vi "Main Page.vi"(8 "error in (no error)":errorcluster, 11 "Node Ptr":T2 format="%.0x") -> (0 "error out":errorcluster)   [LabVIEW 2019, in "OPC UA Client Addon System Explorer.lvlib"]
uses:
  OPC UA Client Addon System Explorer.lvlib
  <vilib>/NI VeriStand/Custom Device API/Custom Device Item Ref.ctl
  Addon Shared/Types/OPCConnection.Properties.ctl
  Addon Shared/SubVIs/Constants.vi
  <vilib>/NI VeriStand/Custom Device API/NI VeriStand - Get Item Property.vi
  <vilib>/NI VeriStand/Custom Device API/Get Item Property (String).vi
  <vilib>/NI VeriStand/Custom Device API/Get Item Property (U16).vi
  <vilib>/NI VeriStand/Custom Device API/Get Item Property (Dependent File).vi
  <vilib>/NI VeriStand/Custom Device API/NI VeriStand - Set Item Property.vi
  <vilib>/NI VeriStand/Custom Device API/Set Item Property (String).vi
  <vilib>/NI VeriStand/Custom Device API/Set Item Property (U16).vi
  <vilib>/Utility/libraryn.llb/Get File Extension.vi
  <vilib>/Utility/MD5Checksum.llb/MD5Checksum File.vi
  <vilib>/NI VeriStand/Custom Device API/Set Item Property (Dependent File).vi
  <vilib>/Utility/libraryn.llb/Check if File or Folder Exists.vi
  <vilib>/NI VeriStand/Custom Device API/NI VeriStand - Remove Item Property.vi
  <vilib>/NI VeriStand/Custom Device API/Custom Device API.lvlib
  Addon Shared/OPC UA Client Addon Shared.lvlib
panel:
  out "Version":string
  in  "Header 2":cluster{"Section Name":string}={"Section Name"="Connection Settings"}
  in  "Login Info":cluster{"User Name":string, "Password":string}
  in  "Security Policy":T1
  in  "Server Certificate":path
  in  "Client Certificate":path
  in  "Server Port":u16=49350
  in  "Server IP Address":string
  in  "SHDocVw.IWebBrowser":refnum<k7>(container)
  in  "Header":cluster{"Section Name":string}={"Section Name"="Custom Device Item Settings"}
  in  "Description":string
  in  "Name":string
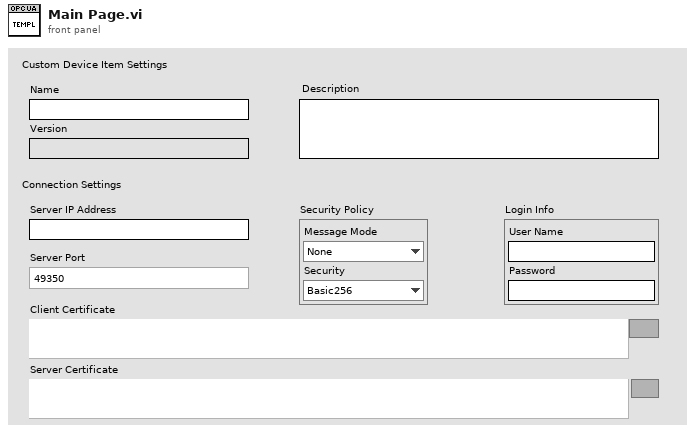
[diagram p1: front panel]
types:
  T1 = cluster{"Message Mode":enum16{"None", "Sign", "Sign and Encrypt"}, "Security":enum16{"Basic256", "Basic128Rsa15"}}
  T2 = typedef "Custom Device API.lvlib/Custom Device Item Ref.ctl" = u64
  T3 = typedef "Custom Device API.lvlib/Custom Device Item Info.ctl" = cluster{"Name":string, "Is Channel":bool, "GUID":string, "Is Waveform":bool}
  T4 = typedef "OPC UA Client Addon Shared.lvlib/OPCConnection.Properties.ctl" = cluster{"Server IP Address":string, "Server Port":u16, "Message Mode":enum16{"None", "Sign", "Sign and Encrypt"}, "Security":enum16{"Basic256", "Basic128Rsa15"}, "User Name":string, "Password":string, "Client Certificate":path, "Server Certificate":path, "Server Certificate (RT)":path, "Client Certificate (RT)":path}
  T5 = typedef "Custom Device API.lvlib/Custom Device Commands.ctl" = enum16{"Default", "Item renamed", "Shutdown", "Dynamic button pressed"}
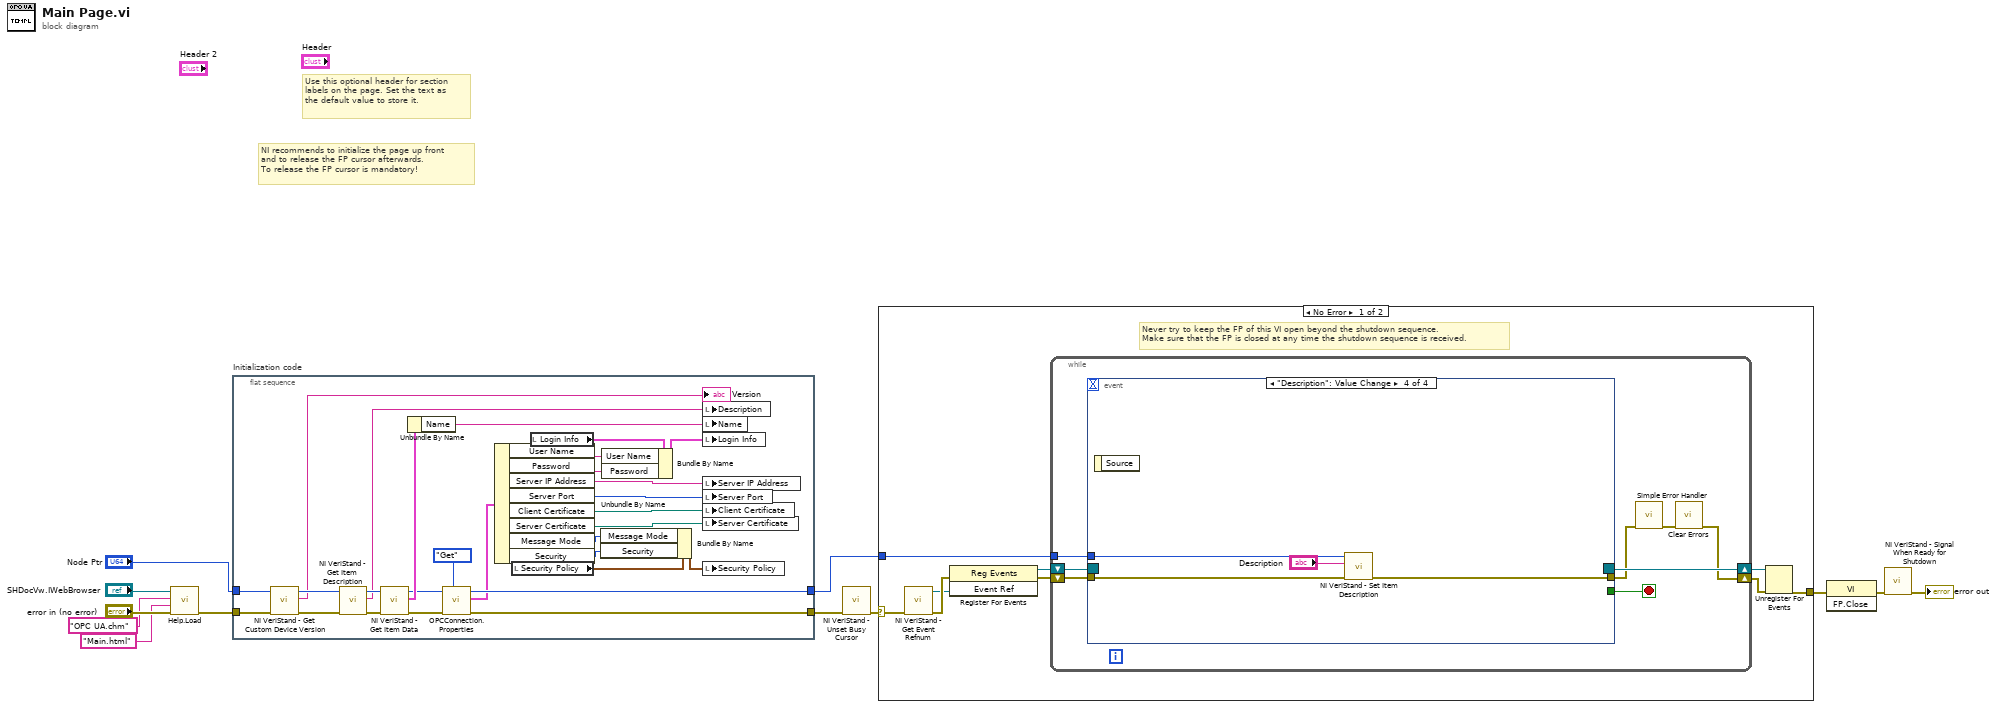
[diagram p0: block diagram]
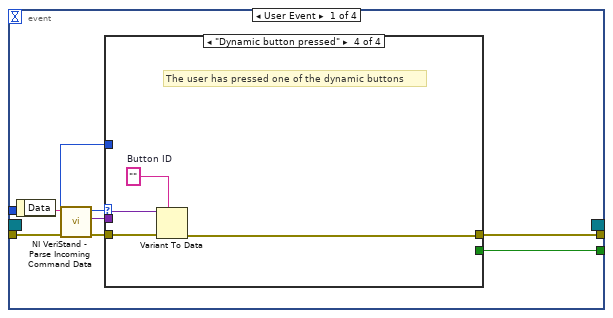
[diagram p2: hidden frame]
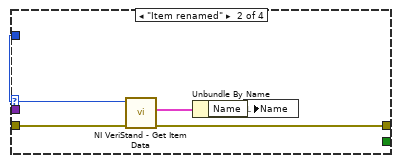
[diagram p4: hidden frame]
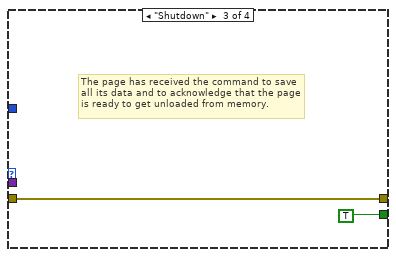
[diagram p5: hidden frame]
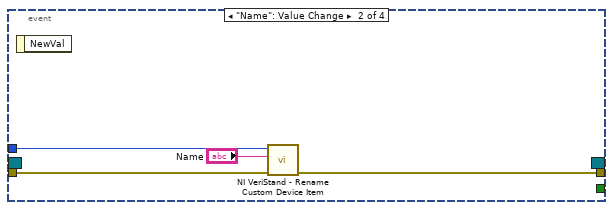
[diagram p6: hidden frame]
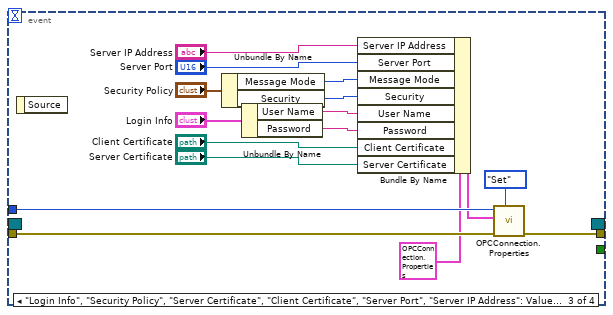
[diagram p7: hidden frame]
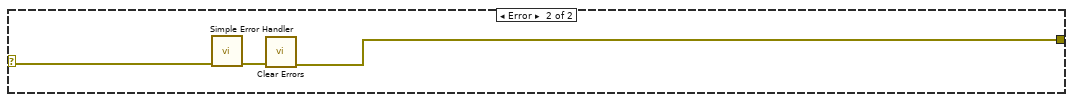
[diagram p8: hidden frame]
diagram:
  # "Use this optional header for section labels on the page. Set the text as the default value to store it."
  # "NI recommends to initialize the page up front\nand to release the FP cursor afterwards.\nTo release the FP cursor is mandatory!"
  n1 = call "Help.Load.vi"("error in (no error)"="error in (no error)", "HTML File"="Main.html" ("Main CHM File"), "Main CHM File"="OPC UA.chm", "SHDocVw.IWebBrowser2"="SHDocVw.IWebBrowser") -> ("error out"=w4:errorcluster)  [unwired: 7 in]
  n2 = flat-sequence "Initialization code" {
    tunnel: w4 -> [w16]
    tunnel: "Node Ptr" -> [w14]
    tunnel: [w33] -> w8
    tunnel: [w31] -> w6
    frame #0 {
      n3 = call <vilib>:"NI VeriStand - Get Custom Device Version.vi"("error in (no error)"=w16, "Device Ref in"=w14) -> ("error out"=w17:errorcluster, "Value"=→"Version":string, "Device Ref out"=w15:T2)  [unwired: 7 in]
      n4 = call <vilib>:"NI VeriStand - Get Item Description.vi"("error in (no error)"=w17, "Item Ref in"=w15) -> ("error out"=w38:errorcluster, "Description"=w39:string, "Item Ref out"=w40:T2)  [unwired: 7 out]
      n5 = call <vilib>:"NI VeriStand - Get Item Data.vi"("error in (no error)"=w38, "Item Ref in"=w40) -> ("error out"=w34:errorcluster, "Item Info"=w37:T3, "Item Ref out"=w32:T2)  [unwired: 7 out]
      n6 = Unbundle By Name(w37) -> ("Name"=w36:string)
      n7 = call "OPCConnection.Properties.vi"("Action"=enum8{"Get", "Set"}."Get", "error in (no error)"=w34, "Item Ref in"=w32) -> ("error out"=w33:errorcluster, "Connection.Properties"=w30:T4, "Item Ref out"=w31:T2)  [unwired: 6 in]
      n8 = Unbundle By Name(w30) -> ("User Name"=w28:string, "Password"=w27:string, "Server IP Address"=w25:string, "Server Port"=w24:u16, "Client Certificate"=w23:path, "Server Certificate"=w22:path, "Message Mode"=w19:enum16{"None", "Sign", "Sign and Encrypt"}, "Security"=w18:enum16{"Basic256", "Basic128Rsa15"})
      n9 = local read "Security Policy"() -> (w20:T1)
      n10 = local read "Login Info"() -> (w29:cluster{"User Name":string, "Password":string})
      n11 = Bundle By Name(cluster=w20, "Message Mode"=w19, "Security"=w18) -> (w21:T1)
      n12 = Bundle By Name(cluster=w29, "User Name"=w28, "Password"=w27) -> (w26:cluster{"User Name":string, "Password":string})
      n13 = local write "Description"(w39) -> ()
      n14 = local write "Name"(w36) -> ()
      n15 = local write "Login Info"(w26) -> ()
      n16 = local write "Server IP Address"(w25) -> ()
      n17 = local write "Server Port"(w24) -> ()
      n18 = local write "Client Certificate"(w23) -> ()
      n19 = local write "Server Certificate"(w22) -> ()
      n20 = local write "Security Policy"(w21) -> ()
    }
  }
  n21 = call <vilib>:"NI VeriStand - Unset Busy Cursor.vi"("error in (no error)"=w8) -> ("error out"=w7:errorcluster)  [unwired: 10 out]
  n22 = case shown="No Error" w7 {
    selector: w7 -> [w41 w104]
    tunnel: [w46 w102] -> w12
    tunnel: w6 -> [w42 _]
    frame No Error {
      # "Never try to keep the FP of this VI open beyond the shutdown sequence.\nMake sure that the FP is closed at any time the shutdown sequence is received."
      n23 = call <vilib>:"NI VeriStand - Get Event Refnum.vi"("error in (no error)"=w41) -> ("error out"=w49:errorcluster, "Event Ref"=w45:refnum<user-event>)  [unwired: 9 out]
      n24 = register-events(error in=w49, w45) -> (reference out=w43:refnum<event-registration>, error out=w44:errorcluster)  [unwired: 1 in]
      n25 = while {
        tunnel: w42 -> [w53]
        shift-right: [w50] -> w47
        shift-left: w44 -> [w56]
        shift-right: [w57] -> w48
        shift-left: w43 -> [w55]
        stop <- w54 stop-if-true
        n26 = event shown="[3] \"Description\": Value Change" {
          selector: w55 -> [_ _ _ _]
          dyn-events: [_ _ _ _] -> w57
          timeout: _ -> [_ _ _ _]
          tunnel: w56 -> [w65 w81 w96 w100]
          tunnel: [w61 _ _ _] -> w54
          tunnel: [w60 w80 w95 w99] -> w52
          tunnel: w53 -> [w59 w79 w94 w101]
          event User Event {
            n27 = event-data() -> ("Data"=w64:string)  [unwired: 1 out]
            n28 = call <vilib>:"NI VeriStand - Parse Incoming Command Data.vi"("error in (no error)"=w65, "Incoming data"=w64) -> ("error out"=w63:errorcluster, "Outgoing data"=w58:variant, "Action"=w62:T5)  [unwired: 7 out]
            n29 = case shown="\"Dynamic button pressed\"" w62 {
              tunnel: w63 -> [w66 w71 w72 w77]
              tunnel: [_ _ TRUE _] -> w61
              tunnel: [w66 w68 w72 w74] -> w60
              tunnel: w59 -> [_ w70 _ _]
              tunnel: w58 -> [_ _ _ w76]
              frame "Default", Default {
              }
              frame "Item renamed" {
                n30 = call <vilib>:"NI VeriStand - Get Item Data.vi"("error in (no error)"=w71, "Item Ref in"=w70) -> ("error out"=w68:errorcluster, "Item Info"=w69:T3)  [unwired: 8 out]
                n31 = Unbundle By Name(w69) -> ("Name"=w67:string)
                n32 = local write "Name"(w67) -> ()
              }
              frame "Shutdown" {
                # "The page has received the command to save all its data and to acknowledge that the page is ready to get unloaded from memory."
              }
              frame "Dynamic button pressed" {
                w75 = ""  # Button ID
                # "The user has pressed one of the dynamic buttons"
                n33 = Variant To Data(error in=w77, type=w75, Variant=w76) -> (error out=w74:errorcluster)  [unwired: 1 out]
              }
            }
          }
          event "Name": Value Change {
            n34 = event-data() -> ()  [unwired: 2 out]
            n35 = call <vilib>:"NI VeriStand - Rename Custom Device Item.vi"("error in (no error)"=w81, "New Name"="Name", "Item Ref in"=w79) -> ("error out"=w80:errorcluster)  [unwired: 1 in, 7 out]
          }
          event "Login Info", "Security Policy", "Server Certificate", "Client Certificate", "Server Port", "Server IP Address": Value Change {
            n36 = event-data() -> ()  [unwired: 2 out]
            n37 = Unbundle By Name("Security Policy") -> ("Message Mode"=w86:enum16{"None", "Sign", "Sign and Encrypt"}, "Security"=w85:enum16{"Basic256", "Basic128Rsa15"})
            n38 = Unbundle By Name("Login Info") -> ("User Name"=w89:string, "Password"=w88:string)
            n39 = Bundle By Name(cluster=T4 {"Server IP Address"="localhost", "Server Port"=49350, "Message Mode"=enum."None", "Security"=enum."Basic256", "User Name"="", "Password"="", "Client Certificate"=path "", "Server Certificate"=path "", "Server Certificate (RT)"=path "", "Client Certificate (RT)"=path ""} ("Connection.Properties"), "Server IP Address"="Server IP Address", "Server Port"="Server Port", "Message Mode"=w86, "Security"=w85, "User Name"=w89, "Password"=w88, "Client Certificate"="Client Certificate", "Server Certificate"="Server Certificate") -> (w82:T4)
            n40 = call "OPCConnection.Properties.vi"("Action"=enum8{"Get", "Set"}."Set", "error in (no error)"=w96, "Connection.Properties"=w82, "Item Ref in"=w94) -> ("error out"=w95:errorcluster)  [unwired: 5 in, 2 out]
          }
          event "Description": Value Change {
            n41 = event-data() -> ()  [unwired: 2 out]
            n42 = call <vilib>:"NI VeriStand - Set Item Description.vi"("error in (no error)"=w100, "Description"="Description", "Item Ref in"=w101) -> ("error out"=w99:errorcluster)  [unwired: 8 out]
          }
        }
        n43 = call <vilib>:"Simple Error Handler.vi"("error in (no error)"=w52) -> ("error out"=w51:errorcluster)  [unwired: 1 in, 7 out]
        n44 = call <vilib>:"Clear Errors.vi"("error in (no error)"=w51) -> ("error out"=w50:errorcluster)  [unwired: 1 in, 5 out]
      }
      n45 = Unregister For Events(event registration refnum=w48, error in=w47) -> (error out=w46:errorcluster)
    }
    frame Error {
      n46 = call <vilib>:"Simple Error Handler.vi"("error in (no error)"=w104) -> ("error out"=w103:errorcluster)  [unwired: 1 in, 7 out]
      n47 = call <vilib>:"Clear Errors.vi"("error in (no error)"=w103) -> ("error out"=w102:errorcluster)  [unwired: 1 in, 5 out]
    }
  }
  n48 = invoke class="VI" method="FP.Close"(error in=w12) -> (error out=w11:errorcluster)  [unwired: 2 in, 2 out]
  n49 = call <vilib>:"NI VeriStand - Signal When Ready for Shutdown.vi"("error in (no error)"=w11) -> ("error out"=→"error out":errorcluster)  [unwired: 10 out]
